vi "Do.vi"(8 "error in (no error)":errorcluster, 10 "Actor in":refnum<class "Actor.lvclass">, 11 "Launch Nested Models Msg":refnum<class "Launch Nested Models Msg.lvclass">) -> (0 "error out":errorcluster, 2 "Actor out":refnum<class "Actor.lvclass">)   [LabVIEW 2015, in "IModel.lvlib" / "Launch Nested Models Msg.lvclass"]
doc: "This VI delivers the message to the actor by calling the appropriate method(s) on the actor."
uses:
  Launch Nested Models Msg.lvclass
  <vilib>/ActorFramework/Actor/Actor.lvclass
  IModel/IModel.lvclass
  Launch Nested Models Msg.lvclass/Launch Nested Models Msg.ctl
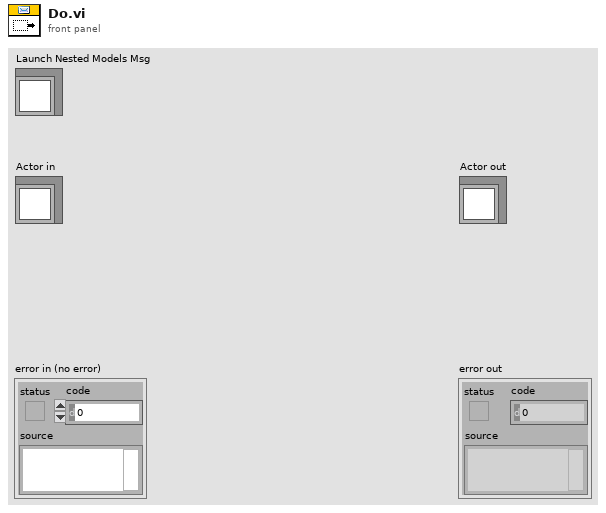
[diagram p1: front panel]
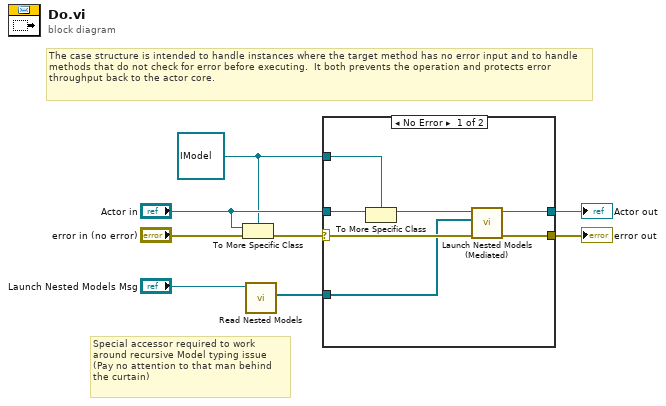
[diagram p0: block diagram]
diagram:
  w3 = refnum<class "IModel.lvclass"> refnum ("Actor in")
  # "Special accessor required to work\naround recursive Model typing issue\n(Pay no attention to that man behind\nthe curtain)"
  # "The case structure is intended to handle instances where the target method has no error input and to handle methods that do not check for error before executing.  It both prevents the operation and protects error throughput back to the actor core."
  n1 = To More Specific Class(target class=w3, reference="Actor in", error in="error in (no error)") -> (error out=w7:errorcluster)  [unwired: 1 out]
  n2 = call "Read Nested Models.vi"("Launch Nested Models Msg"="Launch Nested Models Msg") -> ("Nested Models"=w1:refnum<class "IModel.lvclass">[])  [unwired: 10 in]
  n3 = case shown="No Error" w7 {
    selector: w7 -> [w13 w17]
    tunnel: [w15 w17] -> w6
    tunnel: [w14 w16] -> w5
    tunnel: "Actor in" -> [w12 w16]
    tunnel: w3 -> [w11 _]
    tunnel: w1 -> [w9 _]
    frame No Error {
      n4 = To More Specific Class(target class=w11, reference=w12) -> (specific class reference=w10:refnum<class "IModel.lvclass">)  [unwired: 1 in, 1 out]
      n5 = call-dynamic "Launch Nested Models (Mediated).vi"("error in (no error)"=w13, "Nested Models"=w9, "IModel in"=w10) -> ("error out"=w15:errorcluster, "IModel out"=w14:refnum<class "IModel.lvclass">)  [unwired: 7 in]
    }
    frame Error {
      # "If type check fails, pass the original object out again."
    }
  }
  "error out" <- w6
  "Actor out" <- w5
